vi "overlay helplines.vi"(4 "overlay group":string, 5 "phi0":dbl, 6 "Color":u32(colorbox)=16711680, 7 "#Linien":i32, 8 "error in (no error)":errorcluster, 9 "y0":i32, 10 "x0":i32, 11 "Image":T1) -> (0 "error out":errorcluster, 3 "Image Out":T1)   [LabVIEW 2009, in "POLARIS Vision utility.lvlib"]
uses:
  <vilib>/vision/Image Controls.llb/IMAQ Image.ctl
  <vilib>/Analysis/coordinate.llb/2D Cartesian Coordinate Rotation (Scalar).vi
  POLARIS Vision utility.lvlib
  <vilib>/Analysis/NI_AALPro.lvlib
panel:
  in  "End Point":cluster{"X":i32, "Y":i32}
  in  "Start Point":cluster{"X":i32, "Y":i32}
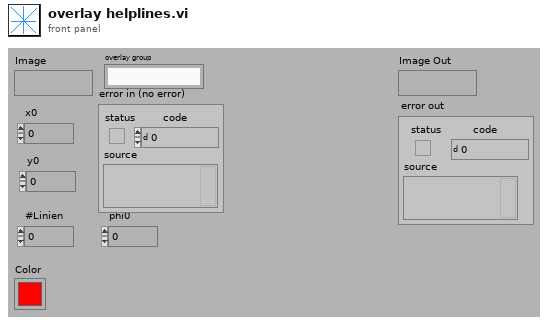
[diagram p1: front panel]
types:
  T1 = typedef "IMAQ Image.ctl" = refnum<image>
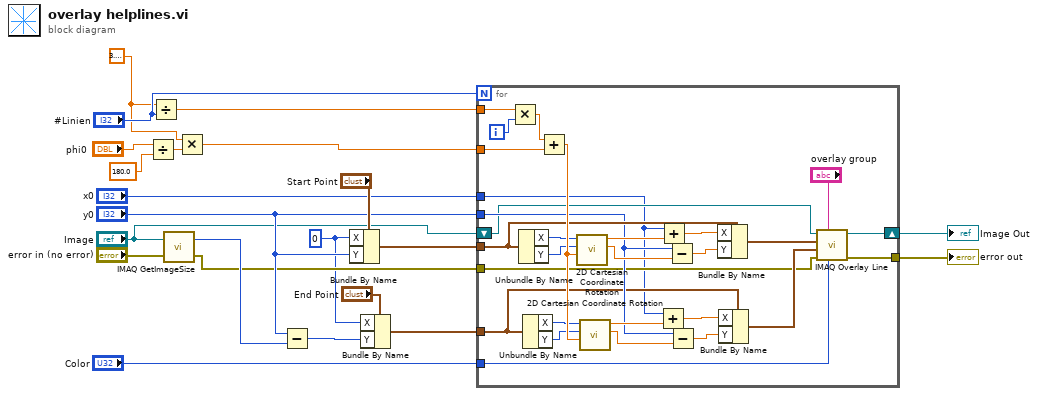
[diagram p0: block diagram]
diagram:
  w1 = 3.141592653589793
  w5 = 0 ("X")
  n1 = Divide(x="phi0", y=180.0 ("x")) -> (x/y=w4:dbl)
  n2 = Divide(x=w1, y="#Linien") -> (x/y=w20:dbl)
  n3 = call "IMAQ GetImageSize"("Image"="Image", "error in (no error)"="error in (no error)") -> ("Y Resolution"=w17:i32, "error out"=w9:errorcluster)  [unwired: 2 in, 1 out]
  n4 = Multiply(x=w1, y=w4) -> (x*y=w2:dbl)
  n5 = Subtract(x="y0", y=w17) -> (x-y=w15:i32)
  n6 = Bundle By Name(cluster="Start Point", "X"=w5, "Y"="y0") -> (w14:cluster{"X":i32, "Y":i32})
  n7 = Bundle By Name(cluster="End Point", "X"=w5, "Y"=w15) -> (w13:cluster{"X":i32, "Y":i32})
  n8 = for {
    N: "#Linien" -> [_]
    tunnel: w20 -> [w51]
    tunnel: w2 -> [w48]
    tunnel: w14 -> [w42]
    tunnel: w13 -> [w29]
    tunnel: "x0" -> [w24]
    tunnel: "y0" -> [w34]
    tunnel: w9 -> [w28]
    tunnel: [w26] -> w7
    tunnel: "Color" -> [w25]
    shift-right: [w27] -> w8
    shift-left: "Image" -> [w32]
    i -> [w50]
    n9 = Multiply(x=w51, y=w50) -> (x*y=w49:dbl)
    n10 = Unbundle By Name(w42) -> ("X"=w46:i32, "Y"=w45:i32)
    n11 = Unbundle By Name(w29) -> ("X"=w44:i32, "Y"=w43:i32)
    n12 = Add(x=w49, y=w48) -> (x+y=w47:dbl)
    n13 = call-poly <vilib>:"2D Cartesian Coordinate Rotation.vi"("theta"=w47, "y"=w45, "x"=w46) -> ("y out"=w40:dbl, "x out"=w41:dbl)  [unwired: 6 in, 1 out]
    n14 = call-poly <vilib>:"2D Cartesian Coordinate Rotation.vi"("theta"=w47, "y"=w43, "x"=w44) -> ("y out"=w33:dbl, "x out"=w35:dbl)  [unwired: 6 in, 1 out]
    n15 = Add(x=w24, y=w35) -> (x+y=w37:dbl)
    n16 = Add(x=w24, y=w41) -> (x+y=w39:dbl)
    n17 = Subtract(x=w34, y=w40) -> (x-y=w38:dbl)
    n18 = Subtract(x=w34, y=w33) -> (x-y=w36:dbl)
    n19 = Bundle By Name(cluster=w42, "X"=w39, "Y"=w38) -> (w31:cluster{"X":i32, "Y":i32})
    n20 = Bundle By Name(cluster=w29, "X"=w37, "Y"=w36) -> (w30:cluster{"X":i32, "Y":i32})
    n21 = call "IMAQ Overlay Line"("Color"=w25, "Group"="overlay group", "error in (no error)"=w28, "End Point"=w30, "Start Point"=w31, "Image"=w32) -> ("error out"=w26:errorcluster, "Image Out"=w27:T1)  [unwired: 4 in]
  }
  "Image Out" <- w8
  "error out" <- w7
